vi "矩形大小（TB）.vi"() -> (11 "point":cluster{"x":i16, "y":i16} caption="大小")   [LabVIEW 2012, in "Picture Box Tools.lvlib"]
uses:
  RectTB.ctl
  Picture Box Tools.lvlib
panel:
  in  "RectTB":T1
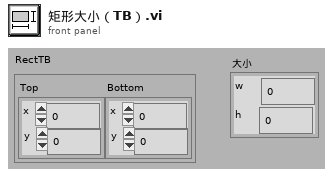
[diagram p1: front panel]
types:
  T1 = typedef "Picture Box Tools.lvlib/RectTB.ctl" = cluster{"Top":cluster{"x":i16, "y":i16}, "Bottom":cluster{"x":i16, "y":i16}}
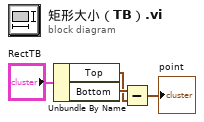
[diagram p0: block diagram]
diagram:
  n1 = Unbundle By Name("RectTB") -> ("Top"=w2:cluster{"x":i16, "y":i16}, "Bottom"=w3:cluster{"x":i16, "y":i16})
  n2 = Subtract(x=w3, y=w2) -> (x-y=→"point":cluster{"x":i16, "y":i16})
